vi "Allow Access to App.vi"(8 "error in (no error)":errorcluster, 11 "URL":string) -> (0 "error out":errorcluster, 3 "LocationURL":string)   [LabVIEW 2016]
panel:
  in  "WebBrowser":refnum<k7>(container)
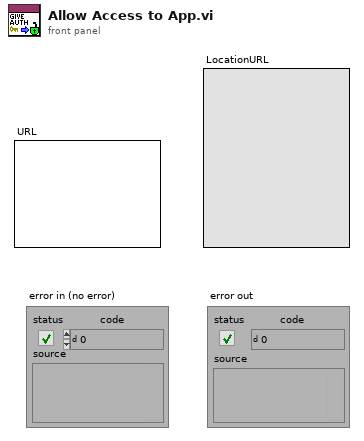
[diagram p1: front panel]
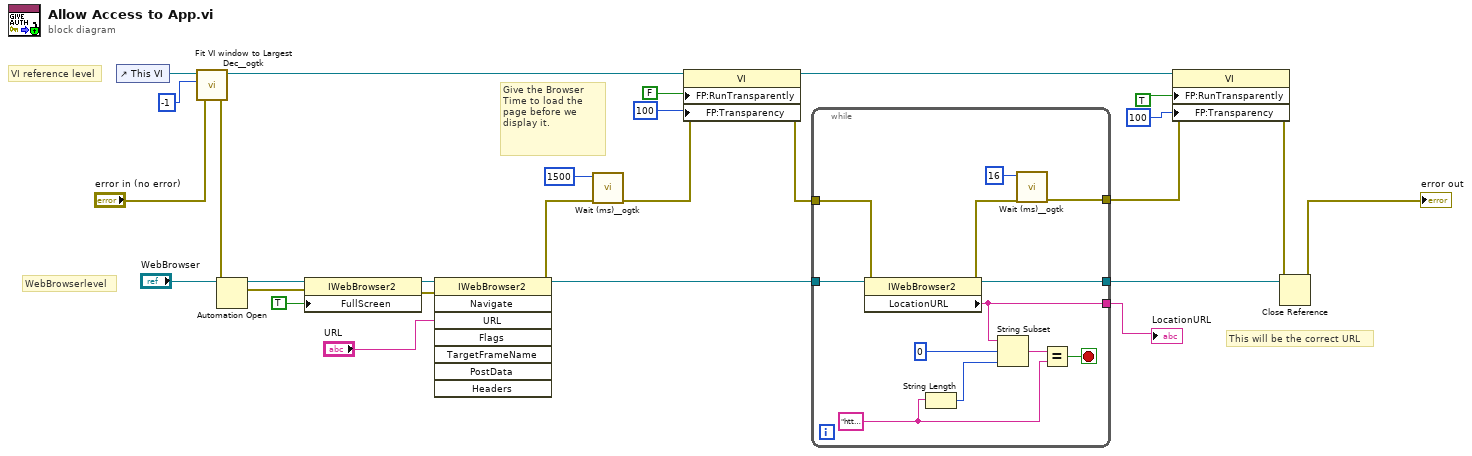
[diagram p0: block diagram]
diagram:
  # "VI reference level"
  # "WebBrowserlevel"
  # "Give the Browser Time to load the page before we display it."
  # "This will be the correct URL"
  n1 = control-ref of="This VI"() -> (w16:refnum<vi>)
  n2 = call <userlib>:"Fit VI window to Largest Dec__ogtk.vi"("error in (no error)"="error in (no error)", "border spacing (2 px)"=-1, "VI Ref (calling VI)"=w16) -> ("error out"=w13:errorcluster, "dup VI Ref"=w15:refnum<vi>)  [unwired: 3 in]
  n3 = Automation Open(error in (no error)=w13, Automation Refnum="WebBrowser") -> (Automation Refnum=w27:refnum<k7>, error out=w12:errorcluster)  [unwired: 2 in]
  n4 = property class="IWebBrowser2"(reference=w27, error in=w12, "FullScreen"=TRUE) -> (reference out=w25:refnum<k7>, error out=w11:errorcluster)
  n5 = invoke class="IWebBrowser2" method="Navigate"(reference=w25, error in=w11, "URL"="URL") -> (reference out=w6:refnum<k7>, error out=w10:errorcluster)  [unwired: 5 in, 6 out]
  n6 = call <userlib>:"Wait (ms)__ogtk.vi"("error in (no error)"=w10, "milliseconds to wait"=u32 1500) -> ("error out"=w9:errorcluster)  [unwired: 8 in, 1 out]
  n7 = property class="VI"(reference=w15, error in=w9, "FP:RunTransparently"=FALSE ("Front Panel Window:Run VI Transparently"), "FP:Transparency"=u8 100 ("Front Panel Window:Transparency")) -> (reference out=w8:refnum<vi>, error out=w5:errorcluster)
  n8 = while {
    tunnel: [w39] -> w7
    tunnel: [w32] -> w22
    tunnel: w6 -> [w31]
    tunnel: w5 -> [w30]
    tunnel: [w28] -> w2
    stop <- w35 stop-if-true
    w33 = "https://login.live.com/oauth20_desktop.srf"
    n9 = property class="IWebBrowser2"(reference=w31, error in=w30) -> (reference out=w39:refnum<k7>, error out=w29:errorcluster, "LocationURL"=w32:string)
    n10 = String Length(string=w33) -> (length=w38:i32)
    n11 = String Subset(string=w32, offset (0)=0, length (rest)=w38) -> (substring=w36:string)
    n12 = call <userlib>:"Wait (ms)__ogtk.vi"("error in (no error)"=w29, "milliseconds to wait"=u32 16) -> ("error out"=w28:errorcluster)  [unwired: 8 in, 1 out]
    n13 = Equal?(x=w36, y=w33) -> (x = y?=w35:bool)
  }
  "LocationURL" <- w22
  n14 = property class="VI"(reference=w8, error in=w2, "FP:RunTransparently"=TRUE ("Front Panel Window:Run VI Transparently"), "FP:Transparency"=u8 100 ("Front Panel Window:Transparency")) -> (error out=w3:errorcluster)  [unwired: 1 out]
  n15 = Close Reference(reference=w7, error in (no error)=w3) -> (error out=→"error out":errorcluster)
